vi "3.2 VelocityControlTest (Geared).vi"(6 "Reset":bool, 7 "Speed (deg/s)":dbl(slide) scale=-700.0..700.0, 10 "Clear Chart":bool, 11 "Stop Button":bool) -> (1 "Speed Chart":T1(graph), 2 "Position Chart":T1(graph))   [LabVIEW 2019, in "SJCube.lvlib"]
uses:
  SJCube.lvlib
  <vilib>/Platform/TimedLoop/XDataNode/XDataNode.xnode
  <vilib>/Platform/TimedLoop/XDataNode/nitl_modes.ctl
  <vilib>/Platform/TimedLoop/XDataNode/XDNodeRunTimeDep.lvlib
  <vilib>/Platform/TimedLoop/XDataNode/wakeup.ctl
  <vilib>/Platform/TimedLoop/XDataNode/timing_clust.ctl
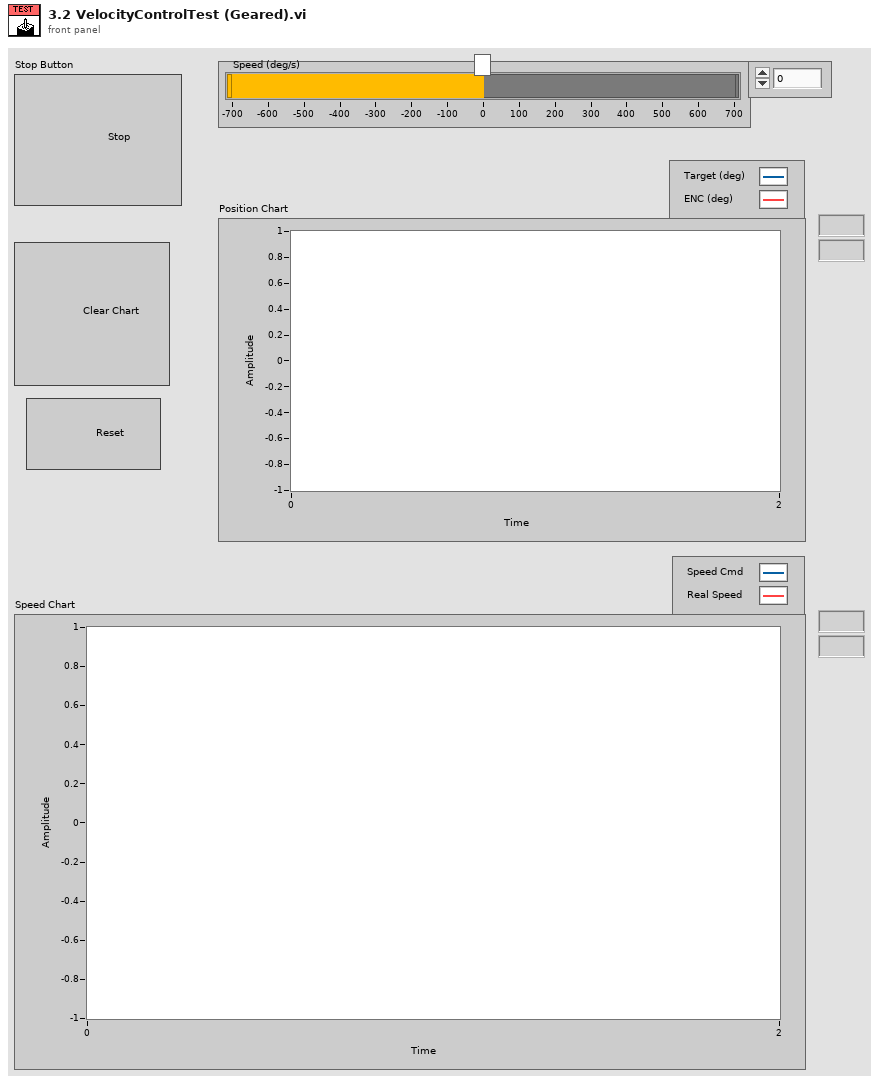
[diagram p1: front panel]
types:
  T1 = cluster{"Position (deg)":dbl, "MotorEncoder (deg)":dbl}
  T2 = typedef "XDNodeRunTimeDep.lvlib/timing_clust.ctl" = cluster{"Expected End [f-1]":u64, "Actual End [f-1]":u64, "Finished Late? [f-1]":bool, "Expected End [i-1]":u64, "Actual End [i-1]":u64, "Finished Late? [i-1]":bool, "Expected Start [i]":u64, "Actual Start [i]":u64, "Expected Start [f]":u64, "Actual Start [f]":u64, "Source Name":string, "Structure Name":string, "Period":i64, "Deadline":i64, "Offset":i64, "Start":i64, "Priority":i32, "Timeout":i32, "Mode":T3, "Wakeup Reason":T4, "Error":errorcluster, "Source Type":string, "Secondary Source Type":string, "Global End Time":u64, "Global Start Time":u64, "Frame Duration":u64, "Iteration Duration":u64, "Assigned CPU":i32, "I/O Scan Engine Mode":u32}
  T3 = typedef "XDNodeRunTimeDep.lvlib/nitl_modes.ctl" = enum32{"No Change", "Process missed periods, maintain original phase", "Discard missed periods, maintain original phase", "Process missed periods, ignore original phase", "Discard missed periods, ignore original phase"}
  T4 = typedef "XDNodeRunTimeDep.lvlib/wakeup.ctl" = enum32{"Normal", "Aborted", "Asynchronous wakeup", "Timing source error", "Timed loop error", "Timeout"}
  T5 = cluster{"Position (deg)":dbl, "MotorEncoder (deg)":dbl}[]
  T6 = cluster{"proportional gain (Kc)":dbl, "integral time (Ti, min)":dbl, "derivative time (Td, min)":dbl}
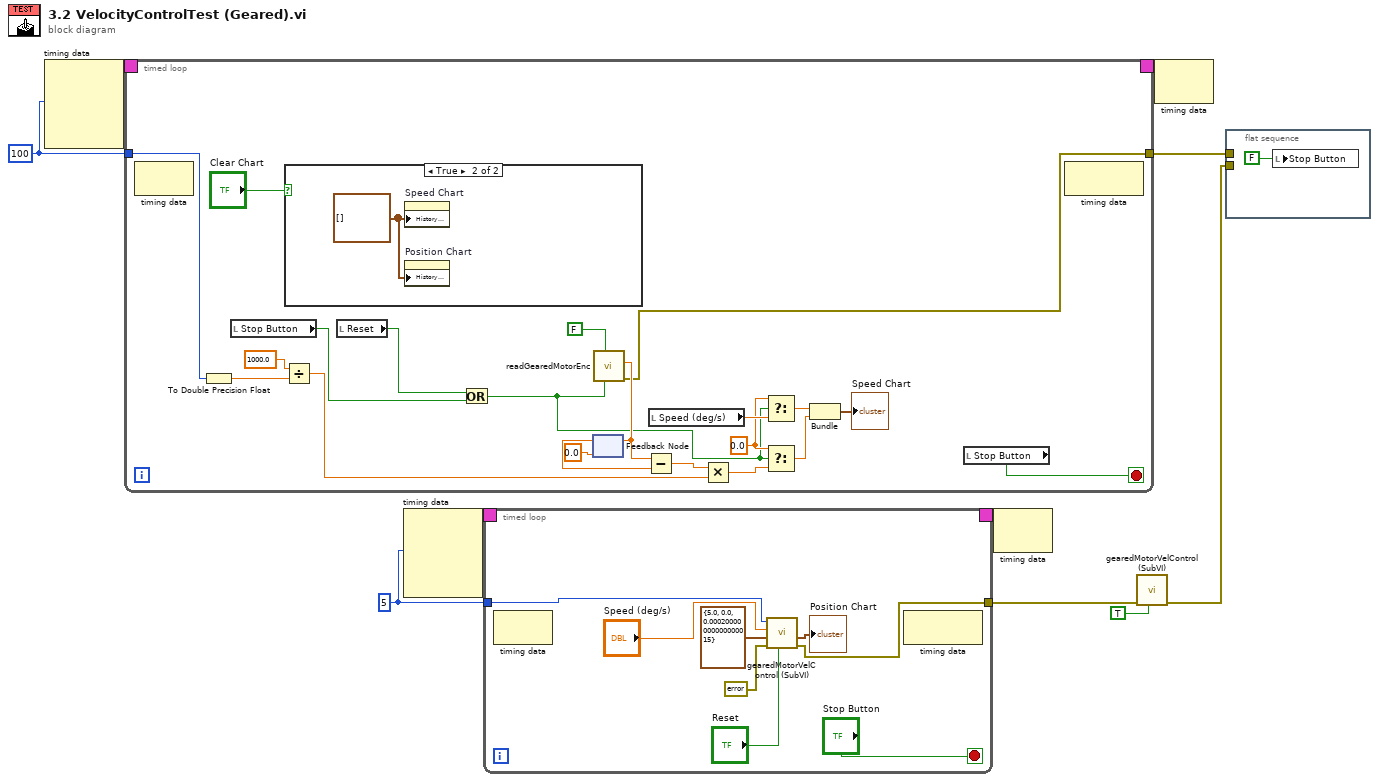
[diagram p0: block diagram]
diagram:
  w3 = i64 100 ("Period")
  w6 = i64 5 ("Period")
  n1 = node-c288(w3) -> (w5:T2)  [unwired: 3 in]
  n2 = timed-loop {
    timing: w5 -> [_]
    timing-out: [_] -> w4
    tunnel: w3 -> [w24]
    tunnel: [w15] -> w1
    stop <- w31 stop-if-true
    w17 = 0.0 ("t")
    n3 = node-c288() -> ()  [unwired: 1 in, 1 out]
    n4 = To Double Precision Float(number=w24) -> (double precision float=w29:dbl)
    n5 = local read "Stop Button"() -> (w13:bool)
    n6 = Divide(x=1000.0, y=w29) -> (x/y=w30:dbl)
    n7 = case shown="True" "Clear Chart" {
      frame False {
      }
      frame True {
        w32 = T5 [] ("History Data")
        n8 = property on="Speed Chart" class="WFChart (strict)"("History Data"=w32) -> ()  [unwired: 2 in, 2 out]
        n9 = property on="Position Chart" class="WFChart (strict)"("History Data"=w32) -> ()  [unwired: 2 in, 2 out]
      }
    }
    n10 = local read "Reset"() -> (w14:bool)
    n11 = Or(x=w14, y=w13) -> (x .or. y?=w12:bool)
    n12 = feedback #1(0.0 ("MotorEncoder (deg)")) -> (w25:dbl)
    n13 = call "readGearedMotorEnc.vi"("Reset Counter"=w12, "Reverse ENC?"=FALSE) -> ("error out"=w15:errorcluster, "gearedMotorEncoder (deg)"=w23:dbl)  [unwired: 8 in]
    n14 = feedback-in #1(w23) -> ()
    n15 = Subtract(x=w23, y=w25) -> (x-y=w27:dbl)
    n16 = local read "Speed (deg/s)"() -> (w20:dbl)
    n17 = Multiply(x=w27, y=w30) -> (x*y=w18:dbl)
    n18 = Select(t=w17, s=w12, f=w20) -> (s? t:f=w19:dbl)
    n19 = Select(t=w17, s=w12, f=w18) -> (s? t:f=w16:dbl)
    n20 = Bundle("Speed (deg/s)"=w19, "t"=w16) -> (→"Speed Chart":cluster{"Speed (deg/s)":dbl, "t":dbl})  [unwired: 1 in]
    n21 = local read "Stop Button"() -> (w31:bool)
    n22 = node-c288() -> ()  [unwired: 1 in, 1 out]
  }
  n23 = node-c288(w6) -> (w10:T2)  [unwired: 3 in]
  n24 = timed-loop {
    timing: w10 -> [_]
    timing-out: [_] -> w9
    tunnel: [w41] -> w8
    tunnel: w6 -> [w37]
    stop <- "Stop Button" stop-if-true
    n25 = node-c288() -> ()  [unwired: 1 in, 1 out]
    n26 = call "gearedMotorVelControl (SubVI).vi"("Reset"="Reset", "error in (no error)"=errorcluster {"status"=FALSE, "code"=0, "source"=""}, "PID gains"=T6 {"proportional gain (Kc)"=5.0, "integral time (Ti, min)"=0.0, "derivative time (Td, min)"=0.00020000000000000015}, "Speed (degs)"="Speed (deg/s)", "dt"=w37) -> ("error out"=w41:errorcluster, "Waveform Chart"=→"Position Chart":T1)  [unwired: 4 in, 1 out]
    n27 = node-c288() -> ()  [unwired: 1 in, 1 out]
  }
  n28 = node-c288(w9) -> ()  [unwired: 1 out]
  n29 = call "gearedMotorVelControl (SubVI).vi"("Reset"=TRUE, "error in (no error)"=w8) -> ("error out"=w2:errorcluster)  [unwired: 7 in, 2 out]
  n30 = node-c288(w4) -> ()  [unwired: 1 out]
  n31 = flat-sequence {
    tunnel: w2 -> [_]
    tunnel: w1 -> [_]
    frame #0 {
      n32 = local write "Stop Button"(FALSE ("Stop Button")) -> ()
    }
  }
